vi "Delay count.vi"(1 "Finished Late? [i-1]":bool) -> (0 "Count":dbl)   [LabVIEW 2018]
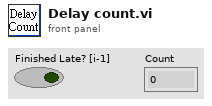
[diagram p1: front panel]
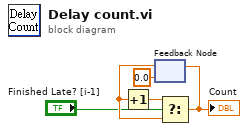
[diagram p0: block diagram]
diagram:
  n1 = feedback #1(0.0) -> (w4:dbl)
  n2 = Increment(x=w4) -> (x+1=w3:dbl)
  n3 = Select(t=w3, s="Finished Late? [i-1]", f=w4) -> (s? t:f=w2:dbl)
  "Count" <- w2
  n4 = feedback-in #1(w2) -> ()
